vi "Close.vi"(8 "error in (no error)":errorcluster, 11 "AI (N Samples) Ref In":T1) -> (0 "error out":errorcluster)   [LabVIEW 2021, in "AI Block.lvlib"]
doc: "Closes the reference to one or more analog input channels, which you use to perform n samples read operations."
uses:
  <vilib>/myRIO/Instrument Drivers/Onboard IO/AI Block/AI Block.lvlib
  <vilib>/myRIO/Instrument Drivers/Onboard IO/AI Block/typedefs/AI Block Reference.ctl
  <vilib>/myRIO/Common/Instrument Driver Framework/Utilities/typedefs/myRIO Generic Hardware Reference.ctl
  <vilib>/myRIO/Common/Instrument Driver Framework/Utilities/typedefs/Hardware Version Enum.ctl
  <vilib>/myRIO/Common/Instrument Driver Framework/Utilities/typedefs/myRIO v1.0 Reference.ctl
  <vilib>/myRIO/Common/Instrument Driver Framework/Utilities/typedefs/Generic FPGA Reference.ctl
  <vilib>/myRIO/Common/Instrument Driver Framework/myRIO v1.0/AI Block/typedefs/AI Block Channels List.ctl
  <vilib>/myRIO/Common/Instrument Driver Framework/myRIO v1.0/AI Block/typedefs/AI Block Channels Enum.ctl
  <vilib>/myRIO/Common/Instrument Driver Framework/Utilities/typedefs/Analog Scaling Constants.ctl
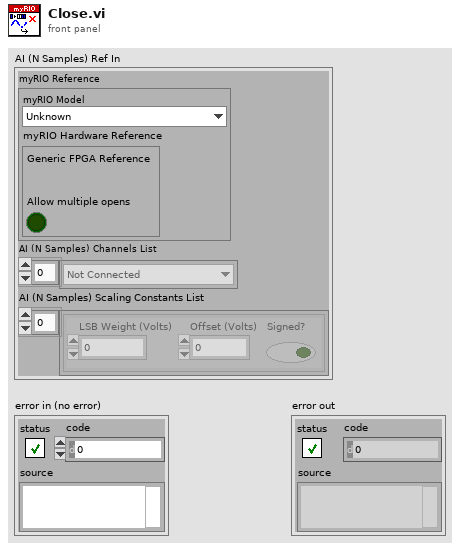
[diagram p1: front panel]
types:
  T1 = typedef "AI Block.lvlib/AI Block Reference.ctl" = cluster{"myRIO Reference":T2, "AI (N Samples) Channels List":T6, "AI (N Samples) Scaling Constants List":T8[]}
  T2 = typedef "myRIO Generic Hardware Reference.ctl" = cluster{"myRIO Model":T3, "myRIO Hardware Reference":T4}
  T3 = typedef "Hardware Version Enum.ctl" = enum16{"Unknown", "myRIO-1900", "myRIO-1950", "roboRIO", "NI ELVIS RIO CM", "ELVIS III"}
  T4 = typedef "myRIO v1.0 Reference.ctl" = cluster{"Generic FPGA Reference":T5, "Allow multiple opens":bool}
  T5 = typedef "Generic FPGA Reference.ctl" = refnum<k20>
  T6 = typedef "AI Block Channels List.ctl" = T7[]
  T7 = typedef "AI Block Channels Enum.ctl" = enum16{"Not Connected", "A/AI0 (N Samples)", "A/AI1 (N Samples)", "A/AI2 (N Samples)", "A/AI3 (N Samples)", "A/AI4 (N Samples)", "A/AI5 (N Samples)", "A/AI6 (N Samples)", "A/AI7 (N Samples)", "A/AI0 (DIFF N Samples)", "A/AI1 (DIFF N Samples)", "A/AI2 (DIFF N Samples)", "A/AI3 (DIFF N Samples)", "B/AI0 (N Samples)", "B/AI1 (N Samples)", "B/AI2 (N Samples)", "B/AI3 (N Samples)", "B/AI4 (N Samples)", "B/AI5 (N Samples)", "B/AI6 (N Samples)", "B/AI7 (N Samples)", "B/AI0 (DIFF N Samples)", "B/AI1 (DIFF N Samples)", "B/AI2 (DIFF N Samples)", "B/AI3 (DIFF N Samples)"}
  T8 = typedef "Analog Scaling Constants.ctl" = cluster{"LSB Weight (Volts)":dbl, "Offset (Volts)":dbl, "Signed?":bool}
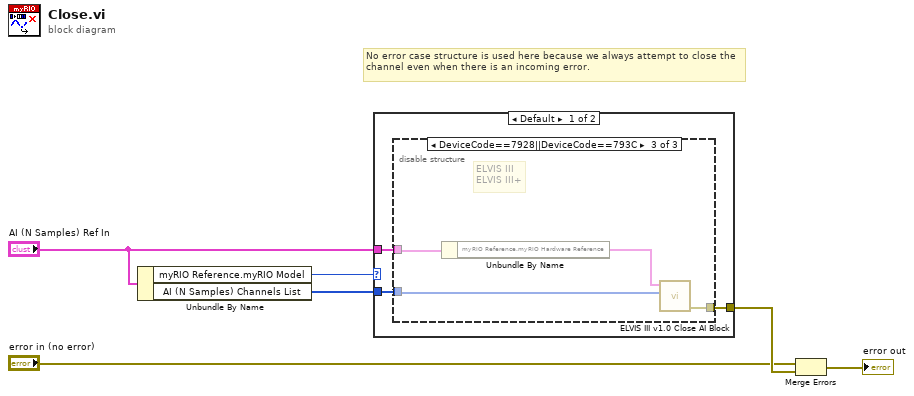
[diagram p0: block diagram]
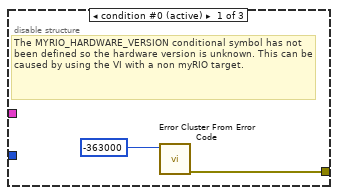
[diagram p2: hidden frame]
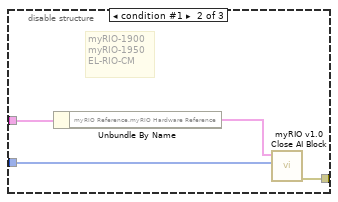
[diagram p3: hidden frame]
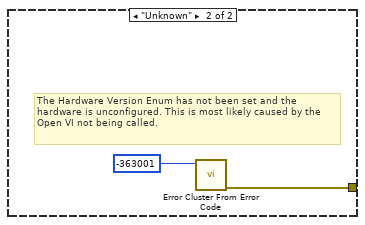
[diagram p4: hidden frame]
diagram:
  # "No error case structure is used here because we always attempt to close the channel even when there is an incoming error."
  n1 = Unbundle By Name("AI (N Samples) Ref In") -> ("myRIO Reference.myRIO Model"=w2:T3, "AI (N Samples) Channels List"=w1:T6)
  n2 = case shown="Default" w2 {
    tunnel: "AI (N Samples) Ref In" -> [w9 _]
    tunnel: [w8 w20] -> w6
    tunnel: w1 -> [w7 _]
    frame Default {
      n3 = disable-structure shown="DeviceCode==7928||DeviceCode==793C" {
        disable-tunnel: w9 -> [_ w15 w18]
        disable-tunnel: [w10 w14 w16] -> w8
        disable-tunnel: w7 -> [_ w12 w17]
        frame condition #0 (active) {
          # "The MYRIO_HARDWARE_VERSION conditional symbol has not been defined so the hardware version is unknown. This can be caused by using the VI with a non myRIO target."
          n4 = call <vilib>:"Error Cluster From Error Code.vi"("error code (0)"=-363000) -> ("error out"=w10:errorcluster)  [unwired: 8 in]
        }
        frame condition #1 {
          # "myRIO-1900\nmyRIO-1950\nEL-RIO-CM"
          n5 = Unbundle By Name(w15) -> ("myRIO Reference.myRIO Hardware Reference"=w13:T4)
          n6 = call <vilib>:"myRIO v1.0 Close AI Block.vi"("AI (N Samples) Channels List"=w12, "myRIO AI (N Samples) Ref In"=w13) -> ("error out"=w14:errorcluster)  [unwired: 9 in]
        }
        frame condition #2 {
          # "ELVIS III\nELVIS III+"
          n7 = Unbundle By Name(w18) -> ("myRIO Reference.myRIO Hardware Reference"=w19:T4)
          n8 = call <vilib>:"ELVIS III v1.0 Close AI Block.vi"("AI (N Samples) Channels List"=w17, "myRIO AI (N Samples) Ref In"=w19) -> ("error out"=w16:errorcluster)  [unwired: 9 in]
        }
      }
    }
    frame "Unknown" {
      # "The Hardware Version Enum has not been set and the hardware is unconfigured. This is most likely caused by the Open VI not being called."
      n9 = call <vilib>:"Error Cluster From Error Code.vi"("error code (0)"=-363001) -> ("error out"=w20:errorcluster)  [unwired: 8 in]
    }
  }
  n10 = Merge Errors("error in (no error)", w6) -> (→"error out":errorcluster)
